vi "Custom_OR.vi"(8 "Input B":bool, 11 "Input A":bool) -> (3 "Output Y":bool)   [LabVIEW 2026]
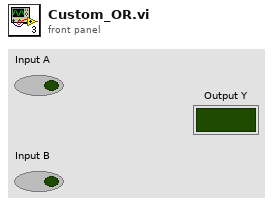
[diagram p1: front panel]
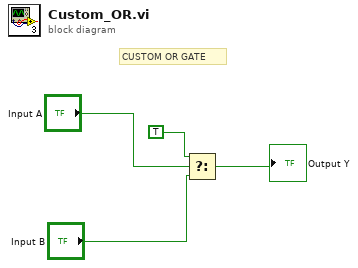
[diagram p0: block diagram]
diagram:
  # "CUSTOM OR GATE"
  n1 = Select(t=TRUE, s="Input A", f="Input B") -> (s? t:f=→"Output Y":bool)
